vi "Imagen_3D_2.vi"() -> ()   [LabVIEW 2016]
uses:
  <vilib>/picture/3D Picture Control/NI_3D Picture Control.lvlib
  <vilib>/Utility/miscctls.llb/LV3DPointTypeDef.ctl
panel:
  in  "Vertical Pointer Slide":dbl(slide) scale=0.0..300.0
  in  "Stop Button":bool
  in  "Camera Position":T1
  out "3D Picture":refnum<vi>(3d-picture)
  in  "Path":path
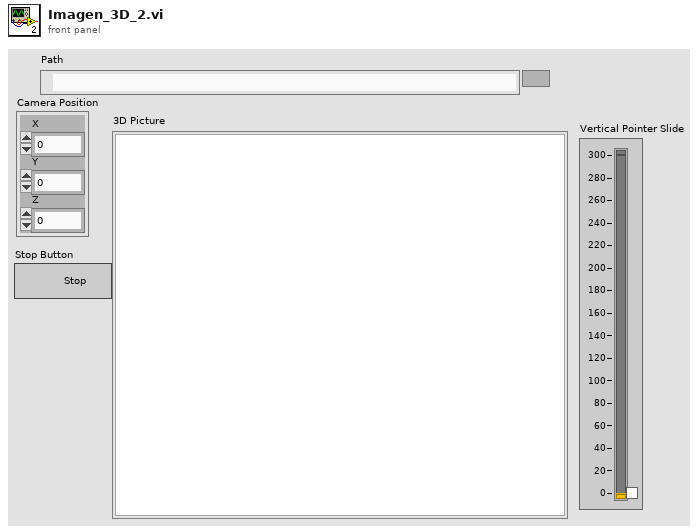
[diagram p1: front panel]
types:
  T1 = typedef "LV3DPointTypeDef.ctl" = cluster{"X":sgl, "Y":sgl, "Z":sgl}
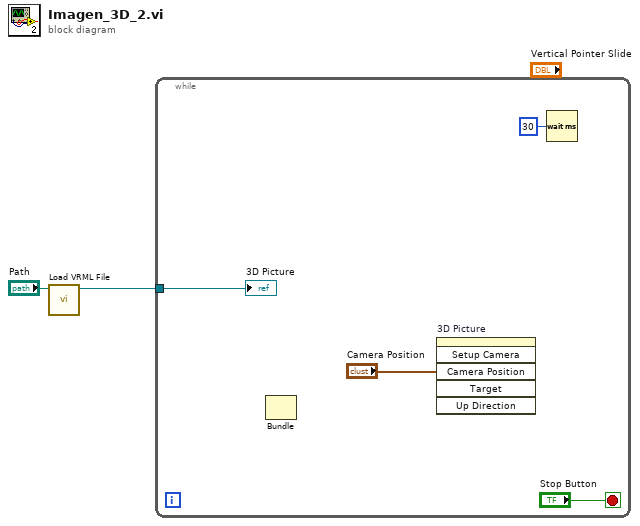
[diagram p0: block diagram]
diagram:
  n1 = call <vilib>:"Load VRML File.vi"("Path"="Path") -> ("Scene:Read Scene File"=w1:refnum<vi>)  [unwired: 9 in, 1 out]
  n2 = while {
    tunnel: w1 -> [w5]
    stop <- "Stop Button" stop-if-true
    n3 = Bundle() -> ()  [unwired: 4 in, 1 out]
    n4 = invoke on="3D Picture" class="SceneGraphDisp (strict)" method="Setup Camera"("Camera Position"="Camera Position") -> ()  [unwired: 5 in, 6 out]
    n5 = Wait (ms)(milliseconds to wait=u32 30) -> ()  [unwired: 1 out]
    "3D Picture" <- w5
  }
